vi "to INT16.vi"(8 "error in":errorcluster, 11 "byte":u8[](array[numeric]) format="%b") -> (0 "error out":errorcluster, 2 "INT16":i16, 3 "remaining bytes":u8[](array[numeric]))   [LabVIEW 2020, in "MessagePack.lvlib" / "MessagePack.lvclass"]
uses:
  MessagePack.lvclass
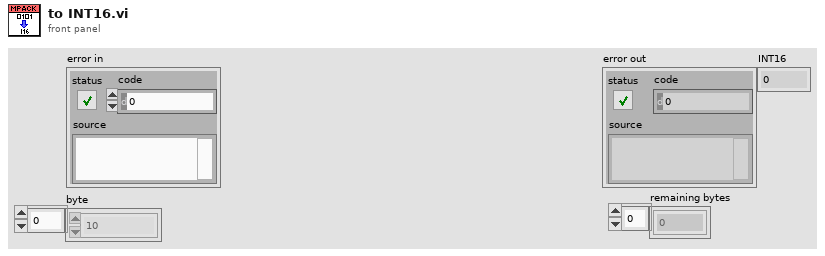
[diagram p1: front panel]
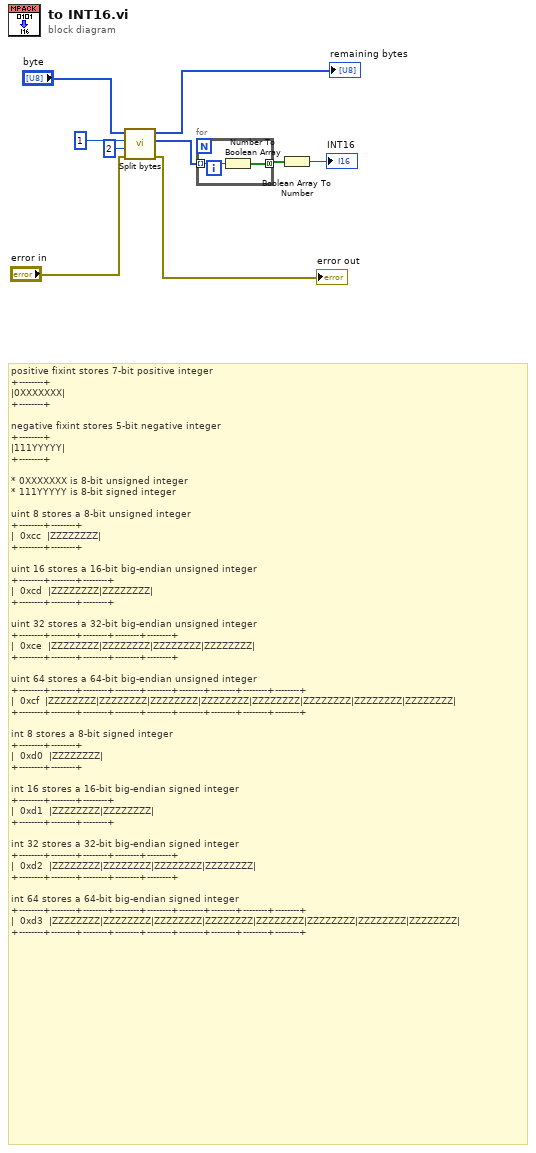
[diagram p0: block diagram]
diagram:
  # "positive fixint stores 7-bit positive integer\n+--------+\n|0XXXXXXX|\n+--------+\n\nnegative fixint stores 5-bit negative integer\n+--------+\n|111YYYYY|\n+--------+\n\n* 0XXXXXXX is 8-bit unsigned integer\n* 111YYYYY is 8-bit signed integer\n\nuint 8 stores a 8-bit unsigned integer\n+--------+--------+\n|  0xcc  |ZZZZZZZZ|\n+--------+--------+\n\nuint 16 stores a 16-bit big-endian unsigned integer\n+--------+--------+--------+\n|  0xcd  |ZZZZZZZZ|ZZZZZZZZ|\n+--------+--------+--------+\n\nuint 32 stores a 32-bit big-endian unsigned integer\n+--------+--------+--------+--------+--------+\n|  0xce  |ZZZZZZZZ|ZZZZZZZZ|ZZZZZZZZ|ZZZZZZZZ|\n+--------+--------+--------+--------+--------+\n\nuint 64 stores a 64-bit big-endian unsigned integer\n+--------+--------+--------+--------+--------+--------+--------+--------+--------+\n|  0xcf  |ZZZZZZZZ|ZZZZZZZZ|ZZZZZZZZ|ZZZZZZZZ|ZZZZZZZZ|ZZZZZZZZ|ZZZZZZZZ|ZZZZZZZZ|\n+--------+--------+--------+--------+--------+--------+--------+--------+--------+\n\nint 8 stores a 8-bit signed integer\n+--------+--------+\n|  0xd0  |ZZZZZZZZ|\n+--------+--------+\n\nint 16 stores a 16-bit big-endian signed integer\n+--------+--------+--------+\n|  0xd1  |ZZZZZZZZ|ZZZZZZZZ|\n+--------+--------+--------+\n\nint 32 stores a 32-bit big-endian signed integer\n+--------+--------+--------+--------+--------+\n|  0xd2  |ZZZZZZZZ|ZZZZZZZZ|ZZZZZZZZ|ZZZZZZZZ|\n+--------+--------+--------+--------+--------+\n\nint 64 stores a 64-bit big-endian signed integer\n+--------+--------+--------+--------+--------+--------+--------+--------+--------+\n|  0xd3  |ZZZZZZZZ|ZZZZZZZZ|ZZZZZZZZ|ZZZZZZZZ|ZZZZZZZZ|ZZZZZZZZ|ZZZZZZZZ|ZZZZZZZZ|\n+--------+--------+--------+--------+--------+--------+--------+--------+--------+"
  n1 = call "Split bytes.vi"("error in"="error in", "End index"=2, "Start index"=1, "bytes in"="byte") -> ("error out"=→"error out":errorcluster, "selected bytes"=w4:u8[], "remaining bytes"=→"remaining bytes":u8[])  [unwired: 4 in, 1 out]
  n2 = for {
    tunnel: w4 -> [w11] mode=indexing
    tunnel: [w10] -> w8 mode=concatenating
    n3 = Number To Boolean Array(number=w11) -> (Boolean array=w10:bool[])
  }
  n4 = Boolean Array To Number(Boolean array=w8) -> (number=→"INT16":i16)
